vi "subDFD_Set Boolean Value by Name.vi"(8 "error in (no error)":errorcluster, 9 "Boolean":bool, 10 "Control Name":string, 11 "vi reference in":refnum<vi>) -> (0 "error out":errorcluster, 3 "vi reference out":refnum<vi>)   [LabVIEW 2023]
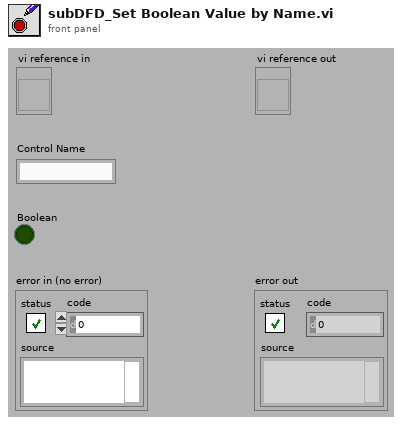
[diagram p1: front panel]
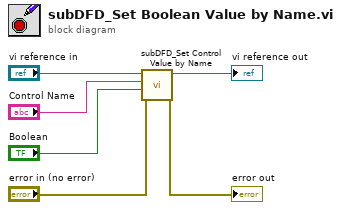
[diagram p0: block diagram]
diagram:
  n1 = call <vilib>:"subDFD_Set Control Value by Name.vi"("error in (no error)"="error in (no error)", "Value"="Boolean", "control name"="Control Name", "vi reference in"="vi reference in") -> ("error out"=→"error out":errorcluster, "vi reference out"=→"vi reference out":refnum<vi>)  [unwired: 6 out]
